vi "Read Input SGL Values.vi"(8 "error in (no error)":errorcluster, 9 "number of registers":u16, 10 "starting address":u16, 11 "device data model in":refnum<class "ICPCON PM3114 Data Model.lvclass">) -> (0 "error out":errorcluster, 2 "data":sgl[](array[numeric]), 3 "device data model out":refnum<class "ICPCON PM3114 Data Model.lvclass">)   [LabVIEW 2021, in "ICPCON PM3114 Data Model.lvclass"]
doc: "Reads N input registers from the device model, starting at register M."
uses:
  ICPCON PM3114 Data Model.lvclass
  ICPCON PM3114 Data Model.lvclass/ICPCON PM3114 Data Model.ctl
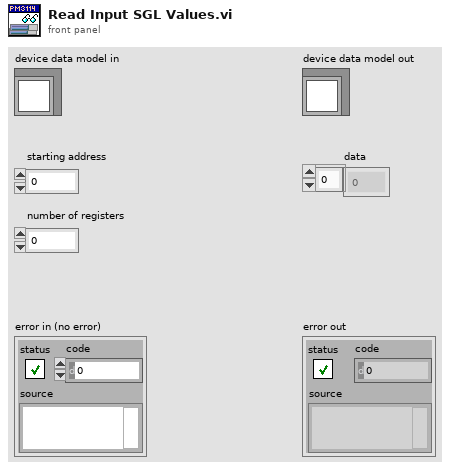
[diagram p1: front panel]
types:
  T1 = typedef "ICPCON PM3114 Data Model.lvclass/Data Model.ctl" = cluster{"UTC":u64, "Power value":sgl[], "ES":u8}
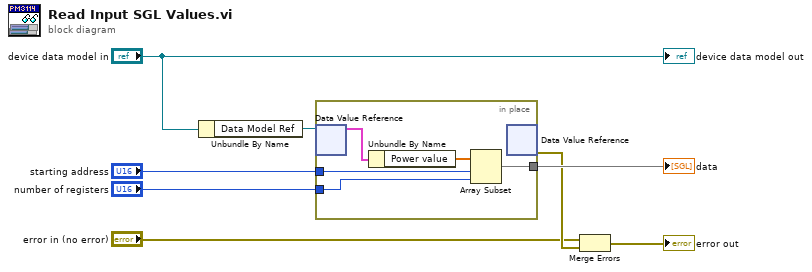
[diagram p0: block diagram]
diagram:
  n1 = Unbundle By Name("device data model in") -> ("Data Model Ref"=w3:refnum<data-value>)
  n2 = in-place {
    in-place-border: "starting address" -> [w10]
    in-place-border: "number of registers" -> [w9]
    in-place-border: [w11] -> w7
    n3 = in-place-dvr #1(w3) -> (w13:T1)  [unwired: 1 out]
    n4 = Unbundle By Name(w13) -> ("Power value"=w12:sgl[])
    n5 = Array Subset(array=w12, index=w10, length=w9) -> (w11:sgl[])
    n6 = in-place-dvr #1() -> (w2:errorcluster)  [unwired: 1 in, 1 out]
  }
  "data" <- w7
  n7 = Merge Errors("error in (no error)", w2) -> (→"error out":errorcluster)
  "device data model out" <- "device data model in"
